vi "Add Context Menu Item.vi"(0 "NotifyIcon in":refnum<class "NotifyIcon.lvclass">, 5 "Item Tag":string, 7 "Item Text":string, 9 "Parent Item Tag (\"\")":string, 11 "error in (no error)":errorcluster, 12 "Item Index (Last)":i32=-1) -> (4 "NotifyIcon out":refnum<class "NotifyIcon.lvclass">, 6 "dub Item Tag":string, 15 "error out":errorcluster)   [LabVIEW 2016, in "NotifyIcon.lvclass"]
doc: "This VI adds a new menu item to the menu. The new menu item will be inserted as a non-default, active and visible item.\nUse the ampersand (&) character in the item text to define the next character as the mnemonic for the Menu Item.\n\n<b>Item Tag</b>\nMust be a unique string that identifies the menu item in the item hierarchy. If this input is left empty the item will not be added to the menu.\n\n<b>Parent Item Tag</b>\nIs used to specify the Tag of the menu item that this item should refer to as its parent. Leaving this input empty or unwired will insert the menu item at the menu root.\n\n<b>Item Index</b>\nWire this input to a numeric value to insert menu items in the middel or top of the menu. Leaving the input unwired inserts the item as the last element under the specified branch (default -1).\n\n\nStinus Olsen\nCIM Industrial Systems A/S\n22. Feb. 2011 15:03\nmailto: seo@cim.as"
uses:
  NotifyIcon.lvclass
  NotifyIcon.lvclass/NotifyIcon.ctl
  System.Windows.Forms
panel:
  # "This VI belongs to the NotifyIcon Toolset. \nA toolset that makes it easy to create, control and manipulate a notification icon in the notification area of the Windows taskbar.\nThe toolset requires Microsoft .NET framework 2.0\n\n\nNOTICE -- YOU MUST LEAVE THIS NOTICE IN PLACE.  PER THE TERMS OF THE LICENSE BELOW, YOU MAY SUBLICENSE THIS SOFTWARE \nIN ANY WAY THAT DOES NOT CONFLICT WITH THIS LICENSE.\n\n### BSD License (http://www.opensource.org/licenses/bsd-license.php) Begin ###\n \nCopyright (c) 2011, Stinus Olsen <seo@cim.as>\n\nAll rights reserved.\n\nRedistribution and use in source and binary forms, with or without modification, are permitted provided that the following conditions are met:\n\n    * Redistributions of source code must retain the above copyright notice, this list of conditions and the following disclaimer.\n    * Redistributions in binary form must reproduce the above copyright notice, this list of conditions and the following disclaimer in the \n       documentation and/or other materials provided with the distribution.\n    * Neither the name of CIM Industrial Systems nor the names of its contributors may be used to endorse or promote products derived \n       from this software without specific prior written permission.\n\nTHIS SOFTWARE IS PROVIDED BY THE COPYRIGHT HOLDERS AND CONTRIBUTORS \"AS IS\" AND ANY EXPRESS OR IMPLIED WARRANTIES, \nINCLUDING, BUT NOT LIMITED TO, THE IMPLIED WARRANTIES OF MERCHANTABILITY AND FITNESS FOR A PARTICULAR PURPOSE ARE \nDISCLAIMED. IN NO EVENT SHALL THE COPYRIGHT OWNER OR CONTRIBUTORS BE LIABLE FOR ANY DIRECT, INDIRECT, INCIDENTAL,\n SPECIAL, EXEMPLARY, OR CONSEQUENTIAL DAMAGES (INCLUDING, BUT NOT LIMITED TO, PROCUREMENT OF SUBSTITUTE GOODS OR \nSERVICES; LOSS OF USE, DATA, OR PROFITS; OR BUSINESS INTERRUPTION) HOWEVER CAUSED AND ON ANY THEORY OF LIABILITY, \nWHETHER IN CONTRACT, STRICT LIABILITY, OR TORT (INCLUDING NEGLIGENCE OR OTHERWISE) ARISING IN ANY WAY OUT OF THE USE \nOF THIS SOFTWARE, EVEN IF ADVISED OF THE POSSIBILITY OF SUCH DAMAGE.\n\n### BSD License End ###"
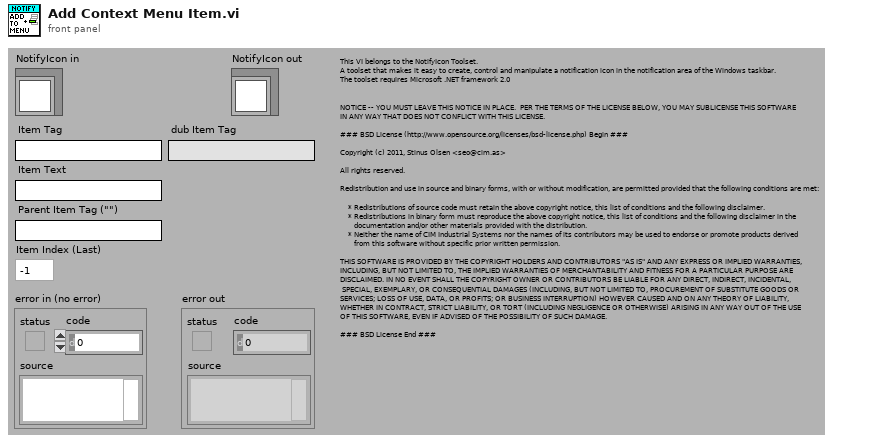
[diagram p1: front panel]
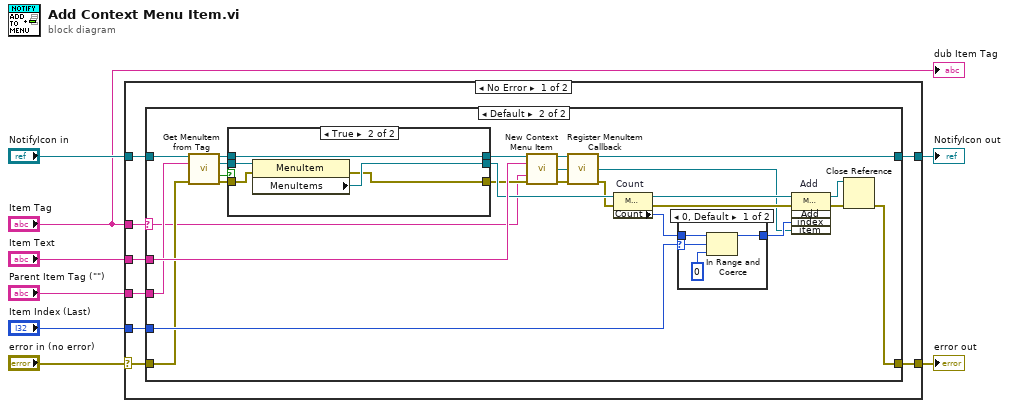
[diagram p0: block diagram]
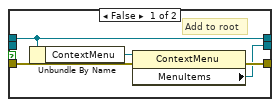
[diagram p3: hidden frame]
diagram:
  n1 = case shown="No Error" "error in (no error)" {
    selector: "error in (no error)" -> [w11 w61]
    tunnel: [w16 w61] -> w7
    tunnel: [w10 w60] -> w5
    tunnel: "NotifyIcon in" -> [w13 w60]
    tunnel: "Parent Item Tag (\"\")" -> [w12 _]
    tunnel: "Item Text" -> [w15 _]
    tunnel: "Item Tag" -> [w9 _]
    tunnel: "Item Index (Last)" -> [w14 _]
    frame No Error {
      n2 = case shown="Default" w9 {
        selector: w9 -> [_ w19]
        tunnel: [w17 w44] -> w16
        tunnel: w15 -> [_ w43]
        tunnel: w14 -> [_ w42]
        tunnel: w13 -> [w18 w41]
        tunnel: w12 -> [_ w40]
        tunnel: w11 -> [w17 w39]
        tunnel: [w18 w22] -> w10
        frame "" {
        }
        frame Default {
          n3 = call "Get MenuItem from Tag.vi"("NotifyIcon in"=w41, "Item Tag"=w40, "error in (no error)"=w39) -> ("NotifyIcon out"=w32:refnum<class "NotifyIcon.lvclass">, "MenuItem"=w29:refnum<k24>, "Found"=w31:bool, "error out"=w30:errorcluster)  [unwired: 9 out]
          n4 = case shown="True" w31 {
            tunnel: w32 -> [w48 w54]
            tunnel: [w48 w54] -> w26
            tunnel: w30 -> [w47 w51]
            tunnel: w29 -> [_ w52]
            tunnel: [w45 w53] -> w28
            tunnel: [w46 w50] -> w27
            frame False {
              # "Add to root"
              n5 = Unbundle By Name(w48) -> ("ContextMenu"=w49:refnum<k24>)
              n6 = property class="ContextMenu"(reference=w49, error in=w47) -> (error out=w46:errorcluster, "MenuItems"=w45:refnum<k24>)  [unwired: 1 out]
            }
            frame True {
              n7 = property class="MenuItem"(reference=w52, error in=w51) -> (error out=w50:errorcluster, "MenuItems"=w53:refnum<k24>)  [unwired: 1 out]
            }
          }
          n8 = call "New Context Menu Item.vi"("NotifyIcon in"=w26, "MenuItem Text"=w43, "MenuItem Tag"=w19, "error in (no error)"=w27) -> ("dub NotifyIcon"=w25:refnum<class "NotifyIcon.lvclass">, "MenuItem"=w24:refnum<k24>, "error out"=w23:errorcluster)  [unwired: 9 out]
          n9 = call "Register MenuItem Callback.vi"("NotifyIcon in"=w25, "MenuItem"=w24, "error in (no error)"=w23) -> ("NotifyIcon out"=w22:refnum<class "NotifyIcon.lvclass">, "dub MenuItem"=w21:refnum<k24>, "error out"=w20:errorcluster)  [unwired: 10 out]
          n10 = property on="Count" class="Menu+MenuItemCollection"(reference=w28, error in=w20) -> (reference out=w36:refnum<k24>, error out=w35:errorcluster, "Count"=w38:i32)
          n11 = case shown="0, Default" w42 {
            selector: w42 -> [w58 _]
            tunnel: w38 -> [w57 w59]
            tunnel: [w55 w59] -> w37
            frame 0, Default {
              n12 = In Range and Coerce(upper limit=w57, x=w58, lower limit=0) -> (coerced(x)=w55:i32)  [unwired: 1 out]
            }
            frame ..-1 {
            }
          }
          n13 = invoke on="Add" class="Menu+MenuItemCollection" method="Add"(reference=w36, error in=w35, "index"=w37, "item"=w21) -> (reference out=w33:refnum<k24>, error out=w34:errorcluster)  [unwired: 1 in, 3 out]
          n14 = Close Reference(reference=w33, error in (no error)=w34) -> (error out=w44:errorcluster)
        }
      }
    }
    frame Error {
    }
  }
  "error out" <- w7
  "NotifyIcon out" <- w5
  "dub Item Tag" <- "Item Tag"
